vi "ArmBegin.vi"(8 "error in (no error)":errorcluster) -> (0 "error out":errorcluster)   [LabVIEW 2020]
doc: "Begin for Arm\n\nInputs:\n -- Error in -- Error cluster -- propagated error input\n--DegreesInCircle--Double--\n--RevolutionsCountPerRotation--Double--\n\nOutputs:\n -- Error out -- Error cluster -- progated error output"
uses:
  <vilib>/Rock Robotics/WPI/ThirdParty/REV Robotics/REVLib/Typedef/Spark MAX Idle Mode.ctl
  <vilib>/Rock Robotics/WPI/ThirdParty/REV Robotics/REVLib/Typedef/Spark MAX Motor Type.ctl
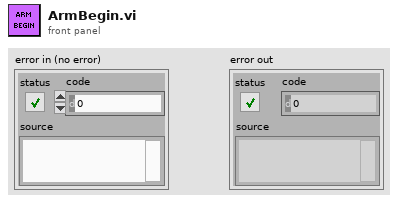
[diagram p1: front panel]
types:
  T1 = typedef "Spark MAX Idle Mode.ctl" = enum16{"Coast", "Brake"}
  T2 = typedef "Spark MAX Motor Type.ctl" = enum16{"Brushed", "Brushless"}
  T3 = typedef "WPI_MotorControlDeviceRef.ctl" = cluster{"DeviceStatus":errorcluster, "Type":T4, "PWM":cluster{"PWM Channel":T5, "DeadBand":T6}, "CAN":cluster{"Device Number":u8, "SetOutput VI Ref":variant, "GetOutput VI Ref":variant, "Enable VI Ref":variant, "Disable VI Ref":variant, "Data":variant}, "Invert":bool, "DIO PWM":cluster{"PWM \"Enable\" Channel":T5, "DIOChannel":T7, "PWM Rate":dbl}}
  T4 = typedef "WPI_MotorControlType.ctl" = enum16{"PWM", "CAN", "DIO PWM"}
  T5 = typedef "FPGA_DIOPWMChannel.ctl" = enum8{"PWM 0", "PWM 1", "PWM 2", "PWM 3", "PWM 4", "PWM 5", "PWM 6", "PWM 7", "PWM 8", "PWM 9", "PWM MXP 0", "PWM MXP 1", "PWM MXP 2", "PWM MXP 3", "PWM MXP 4", "PWM MXP 5", "PWM MXP 6", "PWM MXP 7", "PWM MXP 8", "PWM MXP 9", "Invalid"}
  T6 = typedef "WPI_PWMDeadband.ctl" = cluster{"Name":string, "maxPositivePwm":i32, "minPositivePwm":i32, "centerPwm":i32, "maxNegativePwm":i32, "minNegativePwm":i32, "angularRange":u16}
  T7 = typedef "FPGA_DIOChannel.ctl" = enum8{"DIO 0", "DIO 1", "DIO 2", "DIO 3", "DIO 4", "DIO 5", "DIO 6", "DIO 7", "DIO 8", "DIO 9", "DIO MXP 0", "DIO MXP 1", "DIO MXP 2", "DIO MXP 3", "DIO MXP 4", "DIO MXP 5", "DIO MXP 6", "DIO MXP 7", "DIO MXP 8", "DIO MXP 9", "DIO MXP 10", "DIO MXP 11", "DIO MXP 12", "DIO MXP 13", "DIO MXP 14", "DIO MXP 15", "SPI Port CS1", "SPI Port CS2", "SPI Port CS3", "SPI Port MISO", "SPI Port MOSI", "Invalid"}
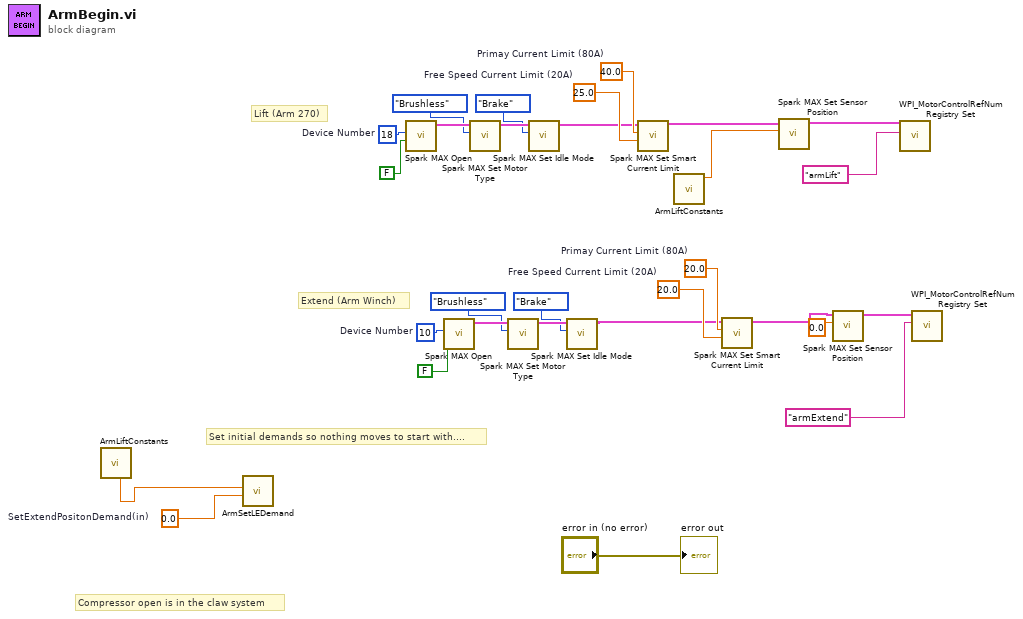
[diagram p0: block diagram]
diagram:
  w4 = 20.0  # Free Speed Current Limit (20A)
  w5 = 20.0  # Primay Current Limit (80A)
  w12 = 0.0  # SetExtendPositonDemand(in)
  w13 = 25.0  # Free Speed Current Limit (20A)
  w14 = 40.0  # Primay Current Limit (80A)
  w21 = u8 18  # Device Number
  w28 = u8 10  # Device Number
  # "Set initial demands so nothing moves to start with...."
  # "Compressor open is in the claw system"
  # "Lift (Arm 270)"
  # "Extend (Arm Winch)"
  n1 = call "ArmLiftConstants.vi"() -> ("Default Angle"=w1:dbl)  [unwired: 8 in, 3 out]
  n2 = call "ArmSetLEDemand.vi"("SetExtendPositonDemand(in)"=w12, "SetLIftPostionDemand(d)"=w1) -> ()  [unwired: 10 in]
  n3 = call <vilib>:"Spark MAX Open.vi"("Invert"=FALSE, "Device Number"=w21) -> ("MotorControlDeviceRef"=w19:T3)  [unwired: 8 in, 1 out]
  n4 = call <vilib>:"Spark MAX Open.vi"("Invert"=FALSE, "Device Number"=w28) -> ("MotorControlDeviceRef"=w26:T3)  [unwired: 8 in, 1 out]
  n5 = call <vilib>:"Spark MAX Set Motor Type.vi"("Motor Type"=Spark_MAX_Motor_Type."Brushless", "MotorControlDevRef"=w19) -> ("MotorControlDeviceRef"=w18:T3)  [unwired: 8 in, 1 out]
  n6 = call <vilib>:"Spark MAX Set Motor Type.vi"("Motor Type"=Spark_MAX_Motor_Type."Brushless", "MotorControlDevRef"=w26) -> ("MotorControlDeviceRef"=w25:T3)  [unwired: 8 in, 1 out]
  n7 = call <vilib>:"Spark MAX Set Idle Mode.vi"("Idle Mode"=Spark_MAX_Idle_Mode."Brake", "MotorControlDeviceRef in"=w18) -> ("MotorControlDeviceRef out"=w11:T3)  [unwired: 8 in, 1 out]
  n8 = call <vilib>:"Spark MAX Set Idle Mode.vi"("Idle Mode"=Spark_MAX_Idle_Mode."Brake", "MotorControlDeviceRef in"=w25) -> ("MotorControlDeviceRef out"=w3:T3)  [unwired: 8 in, 1 out]
  n9 = call <vilib>:"Spark MAX Set Smart Current Limit.vi"("Free Speed Current Limit (20A)"=w13, "Primay Current Limit (80A)"=w14, "MotorControlDeviceRef in"=w11) -> ("MotorControlDeviceRef out"=w9:T3)  [unwired: 7 in, 1 out]
  n10 = call "ArmLiftConstants.vi"() -> ("StartingArmPos"=w6:dbl)  [unwired: 8 in, 3 out]
  n11 = call <vilib>:"Spark MAX Set Smart Current Limit.vi"("Free Speed Current Limit (20A)"=w4, "Primay Current Limit (80A)"=w5, "MotorControlDeviceRef in"=w3) -> ("MotorControlDeviceRef out"=w2:T3)  [unwired: 7 in, 1 out]
  n12 = call <vilib>:"Spark MAX Set Sensor Position.vi"("Position"=w6, "MotorControlDeviceRef"=w9) -> ("MotorControlDeviceRef"=w8:T3)  [unwired: 8 in, 1 out]
  n13 = call <vilib>:"Spark MAX Set Sensor Position.vi"("Position"=0.0, "MotorControlDeviceRef"=w2) -> ("MotorControlDeviceRef"=w7:T3)  [unwired: 8 in, 1 out]
  n14 = call <vilib>:"WPI_MotorControlRefNum Registry Set.vi"("refnum name"="armLift", "MotorControlDevRef"=w8) -> ()  [unwired: 8 in, 2 out]
  n15 = call <vilib>:"WPI_MotorControlRefNum Registry Set.vi"("refnum name"="armExtend", "MotorControlDevRef"=w7) -> ()  [unwired: 8 in, 2 out]
  "error out" <- "error in (no error)"
